vi "Set position 2D (SubVI).vi"(5 "last_pos_xy":cluster{"pos_x":dbl, "pos_y":dbl}, 6 "error in":errorcluster, 7 "Direct":u16(ring) items=["Down", "Up", "Right", "Left"], 8 "Шаг":u32, 9 "VISA Refnum in":refnum<visa-resource-name>="COM7") -> (0 "error out":errorcluster, 2 "set_pos_xy":cluster{"pos_x":dbl, "pos_y":dbl}, 3 "VISA Refnum out":refnum<visa-resource-name>)   [LabVIEW 2018]
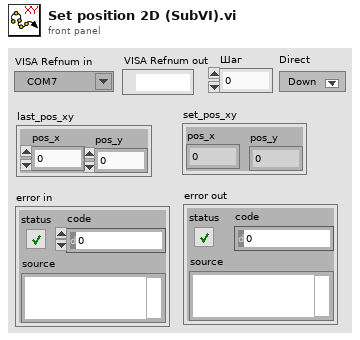
[diagram p1: front panel]
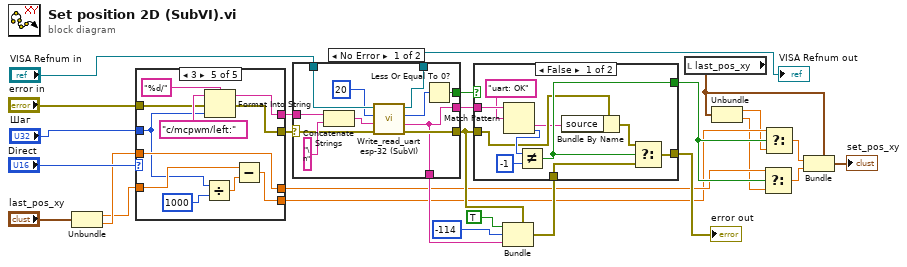
[diagram p0: block diagram]
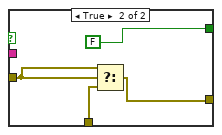
[diagram p2: hidden frame]
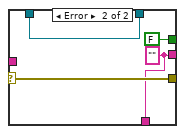
[diagram p3: hidden frame]
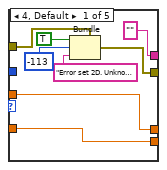
[diagram p4: hidden frame]
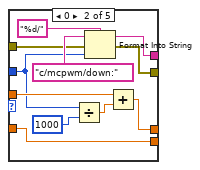
[diagram p5: hidden frame]
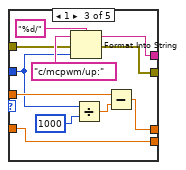
[diagram p6: hidden frame]
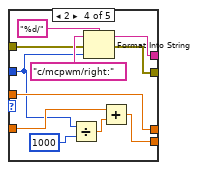
[diagram p7: hidden frame]
diagram:
  n1 = Unbundle("last_pos_xy") -> ("pos_x"=w5:dbl, "pos_y"=w6:dbl)
  n2 = case shown="3" "Direct" {
    tunnel: "Шаг" -> [_ w37 w47 w58 w69]
    tunnel: "error in" -> [w32 w45 w55 w66 w77]
    tunnel: [w31 w43 w54 w65 w76] -> w24
    tunnel: ["" w42 w53 w64 w75] -> w25
    tunnel: w6 -> [w29 w41 w52 w63 w74]
    tunnel: [w29 w40 w51 w63 w74] -> w9
    tunnel: w5 -> [w28 w39 w50 w62 w73]
    tunnel: [w28 w39 w50 w61 w72] -> w8
    frame 4, Default {
      n3 = Bundle(cluster=w32, "status"=TRUE, "code"=-113, "source"="Error set 2D. Unknown direct  ") -> (w31:errorcluster)
    }
    frame 0 {
      n4 = Divide(x=w37, y=u32 1000) -> (x/y=w38:dbl)
      n5 = Format Into String(format string="%d/", initial string="c/mcpwm/down:", error in=w45, w37) -> (resulting string=w42:string, error out=w43:errorcluster)
      n6 = Add(x=w41, y=w38) -> (x+y=w40:dbl)
    }
    frame 1 {
      n7 = Format Into String(format string="%d/", initial string="c/mcpwm/up:", error in=w55, w47) -> (resulting string=w53:string, error out=w54:errorcluster)
      n8 = Divide(x=w47, y=u32 1000) -> (x/y=w48:dbl)
      n9 = Subtract(x=w52, y=w48) -> (x-y=w51:dbl)
    }
    frame 2 {
      n10 = Divide(x=w58, y=u32 1000) -> (x/y=w59:dbl)
      n11 = Format Into String(format string="%d/", initial string="c/mcpwm/right:", error in=w66, w58) -> (resulting string=w64:string, error out=w65:errorcluster)
      n12 = Add(x=w62, y=w59) -> (x+y=w61:dbl)
    }
    frame 3 {
      n13 = Divide(x=w69, y=u32 1000) -> (x/y=w70:dbl)
      n14 = Format Into String(format string="%d/", initial string="c/mcpwm/left:", error in=w77, w69) -> (resulting string=w75:string, error out=w76:errorcluster)
      n15 = Subtract(x=w73, y=w70) -> (x-y=w72:dbl)
    }
  }
  n16 = case shown="No Error" w24 {
    selector: w24 -> [w85 w94]
    tunnel: "VISA Refnum in" -> [w90 w92]
    tunnel: w25 -> [w86 _]
    tunnel: [w84 w94] -> w21
    tunnel: [w80 w91] -> w23
    tunnel: [w82 FALSE] -> w22
    tunnel: [w81 w92] -> w13
    tunnel: [w80 w91] -> w12
    frame No Error {
      n17 = Concatenate Strings(w86, "\n" ("string")) -> (w89:string)
      n18 = call "Write_read_uart esp-32 (SubVI).vi"("error in (no error)"=w85, "write buffer"=w89, "milliseconds to wait"=u32 20, "VISA Refnum in"=w90) -> ("error out 4"=w84:errorcluster, "read buffer"=w80:string, "read bite"=w83:u32, "VISA resource name out"=w81:refnum<visa-resource-name>)
      n19 = Less Or Equal To 0?(x=w83) -> (x <= 0?=w82:bool)
    }
    frame Error {
      w91 = "" ("read buffer")
    }
  }
  "VISA Refnum out" <- w13
  n20 = Bundle(cluster=w21, "status"=TRUE, "code"=-114, "source"=w12) -> (w18:errorcluster)
  n21 = case shown="False" w22 {
    tunnel: w23 -> [w104 _]
    tunnel: w21 -> [w97 w108]
    tunnel: [w99 w106] -> w14
    tunnel: w18 -> [w100 w107]
    tunnel: [w98 FALSE] -> w15
    frame False {
      n22 = Match Pattern(string=w104, regular expression="uart: OK") -> (after substring=w96:string, offset past match=w101:i32)  [unwired: 1 in, 2 out]
      n23 = Not Equal?(x=w101, y=-1 ("offset past match")) -> (x != y?=w98:bool)
      n24 = Bundle By Name(cluster=w97, "source"=w96) -> (w95:errorcluster)
      n25 = Select(t=w95, s=w98, f=w100) -> (s? t:f=w99:errorcluster)
    }
    frame True {
      n26 = Select(t=w108, s=w108, f=w107) -> (s? t:f=w106:errorcluster)
    }
  }
  "error out" <- w14
  n27 = local read "last_pos_xy"() -> (w2:cluster{"pos_x":dbl, "pos_y":dbl})
  n28 = Unbundle(w2) -> ("pos_x"=w4:dbl, "pos_y"=w3:dbl)
  n29 = Select(t=w9, s=w15, f=w3) -> (s? t:f=w10:dbl)
  n30 = Select(t=w8, s=w15, f=w4) -> (s? t:f=w11:dbl)
  n31 = Bundle(cluster=w2, "pos_x"=w11, "pos_y"=w10) -> (→"set_pos_xy":cluster{"pos_x":dbl, "pos_y":dbl})
